vi "ExecuteSkill.vi"(0 "object in":refnum<class "HaltSkill_v2.lvclass">, 2 "Robot in":refnum<class "Robot.lvclass">, 4 "GameRef":refnum<data-value>, 5 "error in (no error)":errorcluster) -> (14 "object out":refnum<class "HaltSkill_v2.lvclass">, 16 "Robot out":refnum<class "Robot.lvclass">, 19 "error out":errorcluster)   [LabVIEW 2023, in "HaltSkill_v2.lvclass"]
uses:
  HaltSkill_v2.lvclass
  Robot_class/Robot.lvclass
  C:/Users/ebert/Documents/codes/SSL/repo/SSL_AI/Object_class/Object.lvclass
  Game_class/Game.lvclass
  Object_class/Object.lvclass/Object.ctl
  Robot_class/Robot.lvclass/Robot.ctl
  Object_class/Read x.vi
  Object_class/Read y.vi
  Robot_class/Read orientation.vi
  Robot_class/Write v_tang.vi
  Robot_class/Write v_norm.vi
  Robot_class/Write v_ang.vi
  Robot_class/Write kick_z.vi
  Robot_class/Write kick_x.vi
  Robot_class/Write dest_x.vi
  Robot_class/Write dest_y.vi
  Robot_class/Write dest_orientation.vi
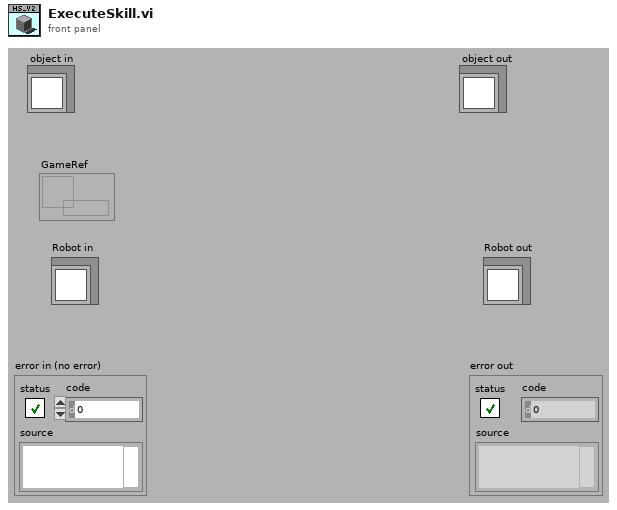
[diagram p1: front panel]
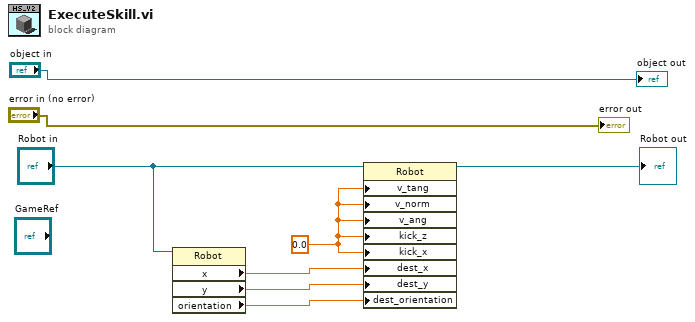
[diagram p0: block diagram]
diagram:
  w5 = 0.0 ("kick_x")
  n1 = property class="Robot"(reference="Robot in") -> ("x"=w8:dbl, "y"=w7:dbl, "orientation"=w6:dbl)  [unwired: 1 in, 2 out]
  n2 = property class="Robot"(reference="Robot in", "v_tang"=w5, "v_norm"=w5, "v_ang"=w5, "kick_z"=w5, "kick_x"=w5, "dest_x"=w8, "dest_y"=w7, "dest_orientation"=w6) -> (reference out=→"Robot out":refnum<class "Robot.lvclass">)  [unwired: 1 in, 1 out]
  "error out" <- "error in (no error)"
  "object out" <- "object in"
